vi "Get FOFB Configuration.vi"(8 "error in (no error)":errorcluster, 9 "TCP Listening Timeout":i32, 10 "Configuration TCP Port":u16, 11 "FOFB Controller IP":string) -> (0 "error out":errorcluster, 3 "FOFB Parameters":T1)   [LabVIEW 2011]
uses:
  Types Definitions/Type FOFB Parameters.ctl
  Types Definitions/Type Network Configuration.ctl
  Types Definitions/Type FA Configuration.ctl
  Types Definitions/Type Acquisition Network Configuration.ctl
  Types Definitions/Type Actuation Network Configuration.ctl
  Types Definitions/Type Configuration Data (GUI to Controller).ctl
  Types Definitions/Type Configuration Change Acknowledge (Controller to GUI).ctl
  Type Definitions.lvlib
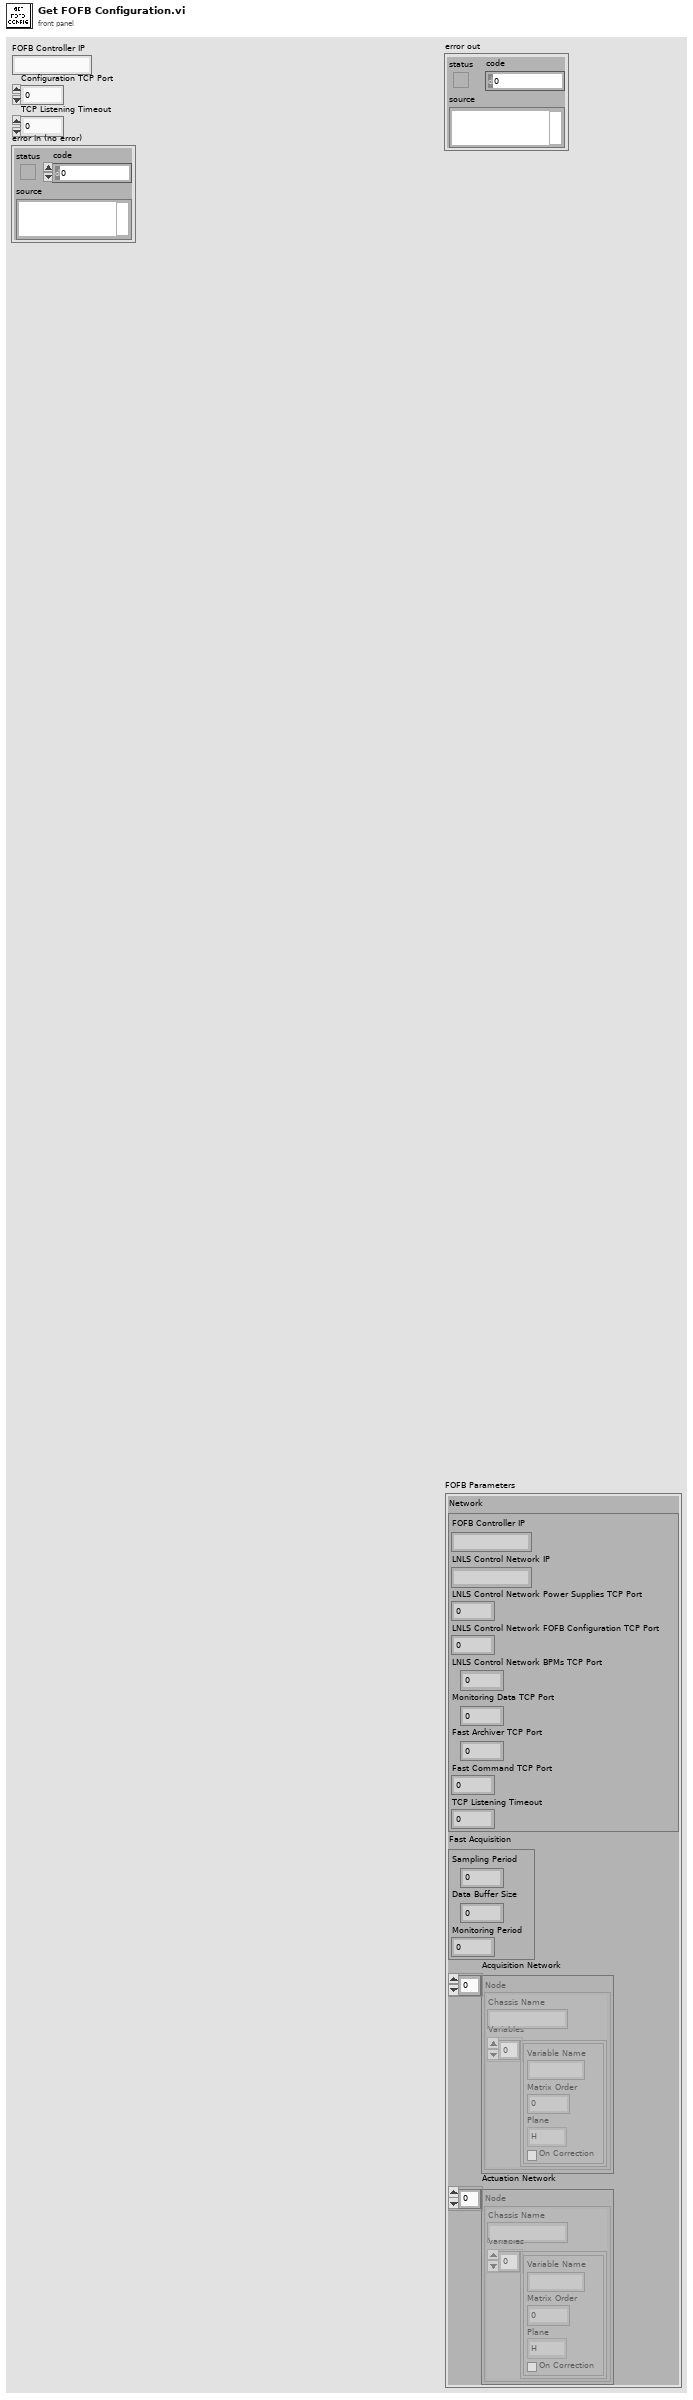
[diagram p1: front panel]
types:
  T1 = typedef "Type Definitions.lvlib/Type FOFB Parameters.ctl" = cluster{"Network":T2, "Fast Acquisition":T3, "Acquisition Network":T4, "Actuation Network":T5}
  T2 = typedef "Type Definitions.lvlib/Type Network Configuration.ctl" = cluster{"FOFB Controller IP":string, "LNLS Control Network IP":string, "LNLS Control Network Power Supplies TCP Port":u16, "LNLS Control Network FOFB Configuration TCP Port":u16, "LNLS Control Network BPMs TCP Port":u16, "Monitoring Data TCP Port":u16, "Fast Archiver TCP Port":u16, "Fast Command TCP Port":u16, "TCP Listening Timeout":i32}
  T3 = typedef "Type Definitions.lvlib/Type FA Configuration.ctl" = cluster{"Sampling Period":u32, "Data Buffer Size":u32, "Monitoring Period":u32}
  T4 = typedef "Type Definitions.lvlib/Type Acquisition Network Configuration.ctl" = cluster{"Chassis Name":string, "Variables":cluster{"Variable Name":string, "Matrix Order":u32, "Plane":enum8{"H", "V"}, "On Correction":bool}[]}[]
  T5 = typedef "Type Definitions.lvlib/Type Actuation Network Configuration.ctl" = cluster{"Chassis Name":string, "Variables":cluster{"Variable Name":string, "Matrix Order":u32, "Plane":enum8{"H", "V"}, "On Correction":bool}[]}[]
  T6 = enum16{"Idle", "Wait Connection", "Read Data", "Process Data", "Write Data", "Close Connection"}
  T7 = typedef "Type Definitions.lvlib/Type Configuration Data (GUI to Controller).ctl" = cluster{"Update Controller Soft Configuration":bool[], "Request RT Execution Trace":string[], "Reference Orbit":dbl[], "Request Response Matrix Folder List":bool[], "Request FOFB Parameters":bool[], "FOFB Parameters":T1[]}
  T8 = typedef "Type Definitions.lvlib/Type Configuration Change Acknowledge (Controller to GUI).ctl" = cluster{"Request Response Matrix List Folder":string[], "FOFB Parameters":T1[]}
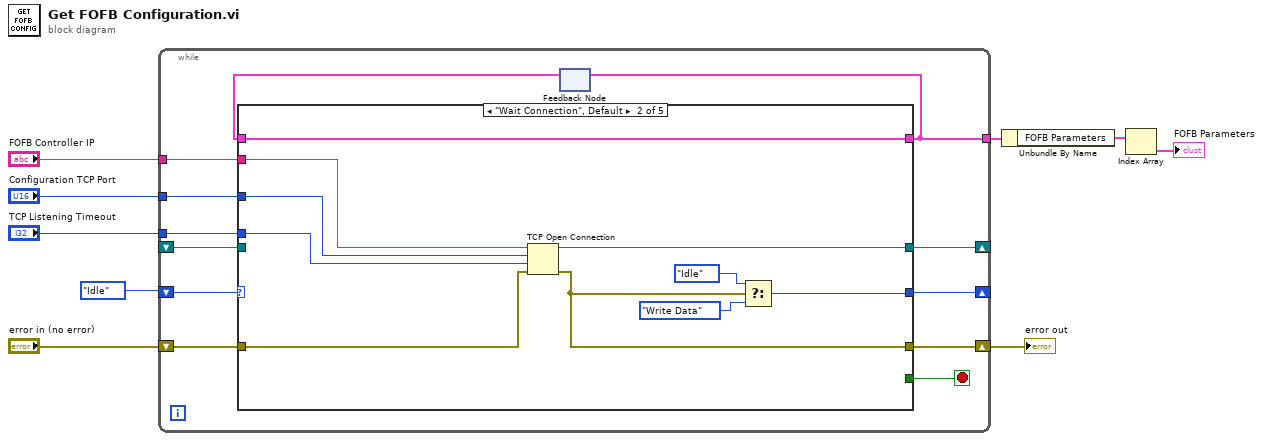
[diagram p0: block diagram]
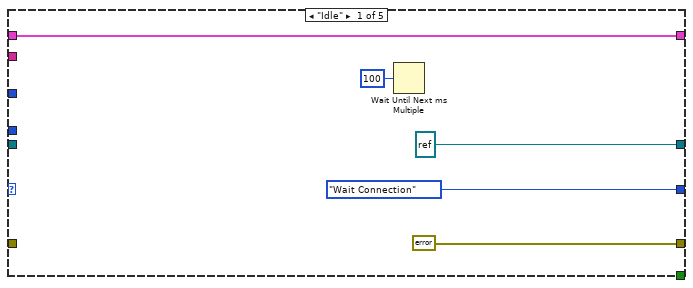
[diagram p2: hidden frame]
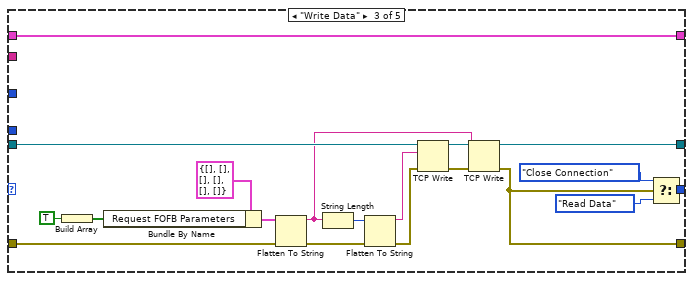
[diagram p3: hidden frame]
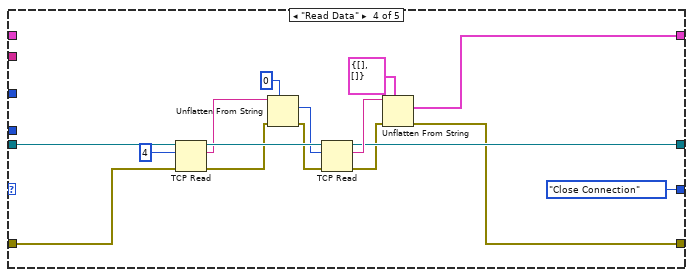
[diagram p4: hidden frame]
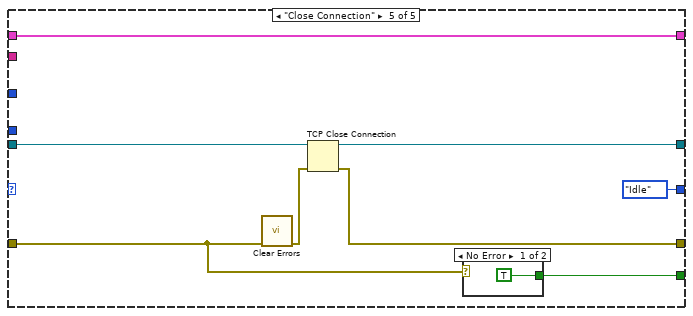
[diagram p5: hidden frame]
diagram:
  n1 = while {
    shift-right: [w21] -> _
    shift-left: T6."Idle" ("f") -> [w20]
    shift-right: [w19] -> _
    shift-left: _ -> [w18]
    tunnel: "FOFB Controller IP" -> [w17]
    tunnel: "Configuration TCP Port" -> [w16]
    tunnel: "TCP Listening Timeout" -> [w15]
    shift-right: [w13] -> w4
    shift-left: "error in (no error)" -> [w14]
    tunnel: [w11] -> w3
    stop <- w10 stop-if-true
    n2 = feedback #1() -> (w12:T8)  [unwired: 1 in]
    n3 = case shown="\"Wait Connection\", Default" w20 {
      tunnel: [refnum<k5> refnum ("connection ID") w33 w55 w64 w79] -> w19
      tunnel: [T6."Wait Connection" ("f") w36 w54 T6."Close Connection" ("f") T6."Idle" ("f")] -> w21
      tunnel: [errorcluster {"status"=FALSE, "code"=0, "source"=""} ("error out") w28 w53 w56 w72] -> w13
      tunnel: w14 -> [_ w32 w51 w63 w74]
      tunnel: w18 -> [_ _ w52 w65 w77]
      tunnel: w17 -> [_ w31 _ _ _]
      tunnel: w16 -> [_ w30 _ _ _]
      tunnel: w15 -> [_ w29 _ _ _]
      tunnel: [w22 w27 w37 w60 w75] -> w11
      tunnel: w12 -> [w22 w27 w37 _ w75]
      tunnel: [_ _ _ _ w73] -> w10
      frame "Idle" {
        n4 = Wait Until Next ms Multiple(millisecond multiple=u32 100) -> ()  [unwired: 1 out]
      }
      frame "Wait Connection", Default {
        n5 = TCP Open Connection(address=w31, remote port or service name=w30, timeout ms (60000)=w29, error in (no error)=w32) -> (connection ID=w33:refnum<k5>, error out=w28:errorcluster)  [unwired: 1 in]
        n6 = Select(t=T6."Idle" ("f"), s=w28, f=T6."Write Data") -> (s? t:f=w36:T6)
      }
      frame "Write Data" {
        n7 = Build Array(TRUE) -> (w40:bool[])
        n8 = Bundle By Name(cluster=T7 {"Update Controller Soft Configuration"=[], "Request RT Execution Trace"=[], "Reference Orbit"=[], "Request Response Matrix Folder List"=[], "Request FOFB Parameters"=[], "FOFB Parameters"=[]} ("Configuration Data (GUI to Controller)"), "Request FOFB Parameters"=w40) -> (w41:T7)
        n9 = Flatten To String(anything=w41, error in (no error)=w51) -> (data string=w46:string, error out=w43:errorcluster)  [unwired: 2 in, 1 out]
        n10 = String Length(string=w46) -> (length=w48:i32)
        n11 = Flatten To String(anything=w48, error in (no error)=w43) -> (data string=w47:string, error out=w42:errorcluster)  [unwired: 2 in, 1 out]
        n12 = TCP Write(connection ID=w52, data in=w47, error in (no error)=w42) -> (connection ID out=w50:refnum<k5>, error out=w49:errorcluster)  [unwired: 2 out]
        n13 = TCP Write(connection ID=w50, data in=w46, error in (no error)=w49) -> (connection ID out=w55:refnum<k5>, error out=w53:errorcluster)  [unwired: 2 out]
        n14 = Select(t=T6."Close Connection" ("f"), s=w53, f=T6."Read Data") -> (s? t:f=w54:T6)
      }
      frame "Read Data" {
        n15 = TCP Read(connection ID=w65, bytes to read=4, error in (no error)=w63) -> (connection ID out=w71:refnum<k5>, data out=w69:string, error out=w59:errorcluster)  [unwired: 2 in]
        n16 = Unflatten From String(type=0 ("bytes to read"), binary string=w69, error in (no error)=w59) -> (value=w67:i32, error out=w61:errorcluster)  [unwired: 2 in, 1 out]
        n17 = TCP Read(connection ID=w71, bytes to read=w67, error in (no error)=w61) -> (connection ID out=w64:refnum<k5>, data out=w66:string, error out=w58:errorcluster)  [unwired: 2 in]
        n18 = Unflatten From String(type=T8 {"Request Response Matrix List Folder"=[], "FOFB Parameters"=[]} ("Configuration Change Acknowledge (Controller to GUI)"), binary string=w66, error in (no error)=w58) -> (value=w60:T8, error out=w56:errorcluster)  [unwired: 2 in, 1 out]
      }
      frame "Close Connection" {
        n19 = call <vilib>:"Clear Errors.vi"("error in (no error)"=w74) -> ("error out"=w78:errorcluster)  [unwired: 6 in]
        n20 = TCP Close Connection(connection ID=w77, error in (no error)=w78) -> (connection ID out=w79:refnum<k5>, error out=w72:errorcluster)  [unwired: 1 in]
        n21 = case shown="No Error" w74 {
          tunnel: [TRUE _] -> w73
          frame No Error {
          }
          frame Error {
          }
        }
      }
    }
    n22 = feedback-in #1(w11) -> ()
  }
  "error out" <- w4
  n23 = Unbundle By Name(w3) -> ("FOFB Parameters"=w2:T1[])
  n24 = Index Array(array=w2) -> (element=→"FOFB Parameters":T1)  [unwired: 1 in]
